vi "color_sensor.vi"() -> ()   [LabVIEW 2022 SP3]
uses:
  <vilib>/DAQmx/read.llb/DAQmx Read (Analog DBL 1Chan 1Samp).vi
  <vilib>/DAQmx/write.llb/DAQmx Write (Digital Bool 1Line 1Point).vi
  <vilib>/DAQmx/create/channels.llb/DAQmx Create Channel (DO-Digital Output).vi
  <vilib>/DAQmx/create/channels.llb/DAQmx Create Channel (AI-Voltage-Basic).vi
  <vilib>/DAQmx/miscellaneous.llb/DAQmx Fill In Error Info.vi
panel:
  out "READ VALUE":dbl
  in  "READ":tag
  in  "Blue Channel":tag
  in  "Green Channel":tag
  in  "Red Channel":tag
  in  "stop":bool
  out "green":bool
  out "blue":bool
  out "red":bool
  out "Numeric":i32
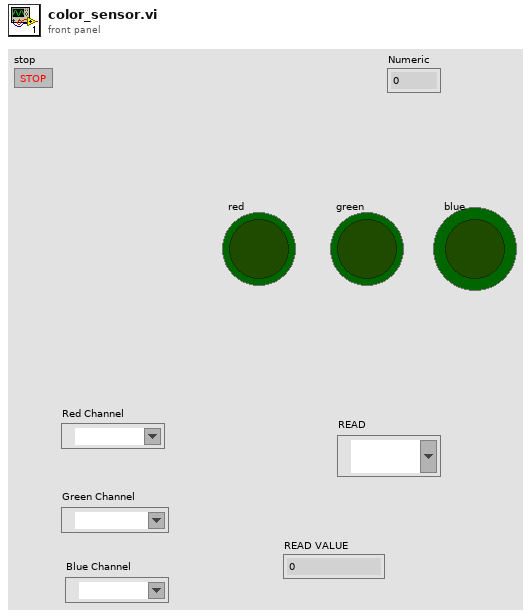
[diagram p1: front panel]
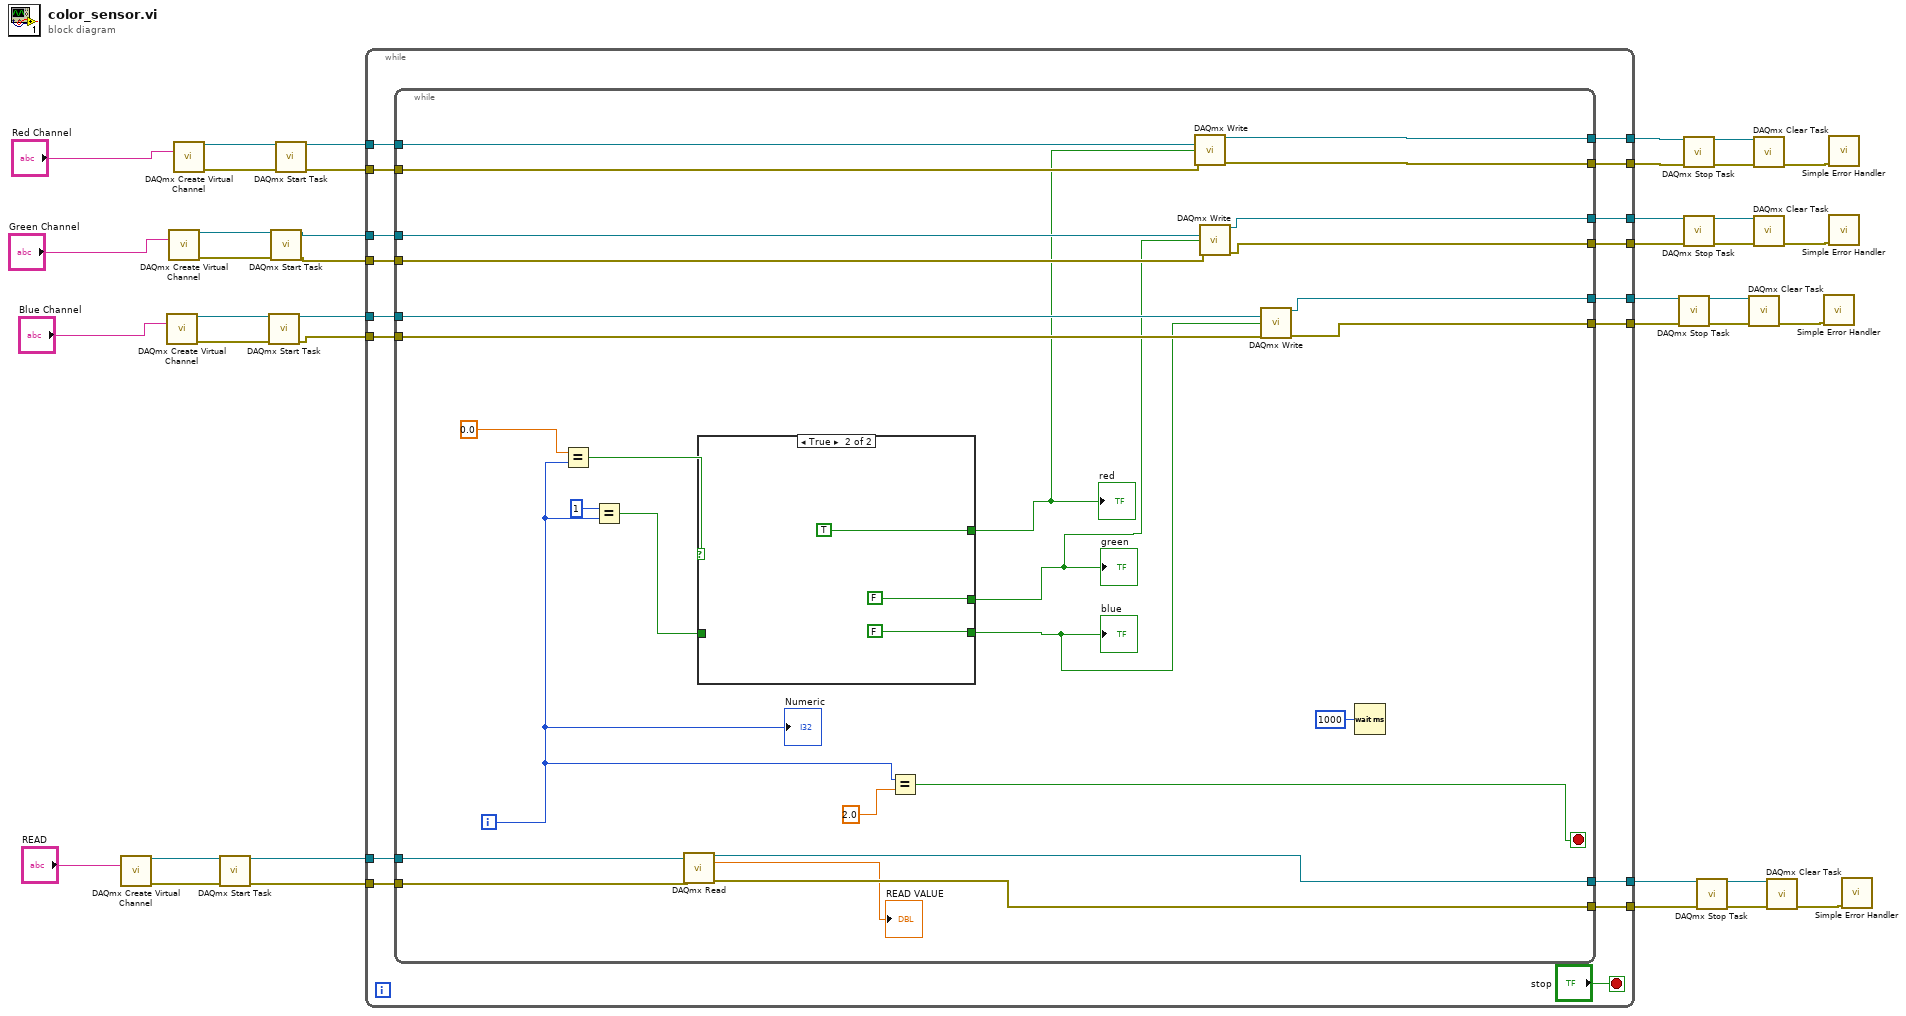
[diagram p0: block diagram]
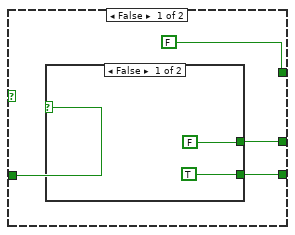
[diagram p2: hidden frame]
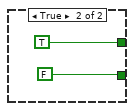
[diagram p3: hidden frame]
diagram:
  n1 = call-poly <vilib>:"DAQmx Create Virtual Channel.vi"("physical channels"="READ") -> ("task out"=w9:refnum<k21>, "error out"=w10:errorcluster)  [unwired: 13 in]
  n2 = call-poly <vilib>:"DAQmx Create Virtual Channel.vi"("lines"="Blue Channel") -> ("task out"=w21:refnum<k21>, "error out"=w22:errorcluster)  [unwired: 13 in]
  n3 = call-poly <vilib>:"DAQmx Create Virtual Channel.vi"("lines"="Green Channel") -> ("task out"=w30:refnum<k21>, "error out"=w31:errorcluster)  [unwired: 13 in]
  n4 = call-poly <vilib>:"DAQmx Create Virtual Channel.vi"("lines"="Red Channel") -> ("task out"=w39:refnum<k21>, "error out"=w40:errorcluster)  [unwired: 13 in]
  n5 = call <vilib>:"DAQmx Start Task.vi"("task/channels in"=w9, "error in"=w10) -> ("task out"=w7:refnum<k21>, "error out"=w6:errorcluster)  [unwired: 12 in]
  n6 = call <vilib>:"DAQmx Start Task.vi"("task/channels in"=w21, "error in"=w22) -> ("task out"=w20:refnum<k21>, "error out"=w19:errorcluster)  [unwired: 12 in]
  n7 = call <vilib>:"DAQmx Start Task.vi"("task/channels in"=w30, "error in"=w31) -> ("task out"=w29:refnum<k21>, "error out"=w28:errorcluster)  [unwired: 12 in]
  n8 = call <vilib>:"DAQmx Start Task.vi"("task/channels in"=w39, "error in"=w40) -> ("task out"=w38:refnum<k21>, "error out"=w37:errorcluster)  [unwired: 12 in]
  n9 = while {
    tunnel: w38 -> [w56]
    tunnel: w37 -> [w55]
    tunnel: [w54] -> w33
    tunnel: [w53] -> w32
    tunnel: w29 -> [w52]
    tunnel: w28 -> [w51]
    tunnel: [w50] -> w24
    tunnel: [w49] -> w23
    tunnel: w20 -> [w48]
    tunnel: w19 -> [w47]
    tunnel: [w46] -> w15
    tunnel: [w45] -> w14
    tunnel: w7 -> [w44]
    tunnel: w6 -> [w43]
    tunnel: [w42] -> w2
    tunnel: [w41] -> w1
    stop <- "stop" stop-if-true
    n10 = while {
      tunnel: w56 -> [w77]
      tunnel: w55 -> [w76]
      tunnel: [w75] -> w54
      tunnel: [w74] -> w53
      tunnel: w52 -> [w73]
      tunnel: w51 -> [w72]
      tunnel: [w71] -> w50
      tunnel: [w70] -> w49
      tunnel: w48 -> [w69]
      tunnel: w47 -> [w68]
      tunnel: [w67] -> w46
      tunnel: [w66] -> w45
      tunnel: w44 -> [w62]
      tunnel: w43 -> [w61]
      tunnel: [w60] -> w42
      tunnel: [w59] -> w41
      i -> [w79]
      stop <- w84 stop-if-true
      n11 = Equal?(x=0.0, y=w79) -> (x = y?=w81:bool)
      n12 = Equal?(x=1, y=w79) -> (x = y?=w80:bool)
      n13 = call-poly <vilib>:"DAQmx Read.vi"("task/channels in"=w62, "error in"=w61) -> ("task out"=w60:refnum<k21>, "data"=→"READ VALUE":dbl, "error out"=w59:errorcluster)  [unwired: 11 in]
      n14 = case shown="True" w81 {
        tunnel: [FALSE TRUE] -> w65
        tunnel: w80 -> [w89 _]
        tunnel: [w87 FALSE] -> w64
        tunnel: [w86 FALSE] -> w63
        frame False {
          n15 = case shown="False" w89 {
            tunnel: [FALSE TRUE] -> w87
            tunnel: [TRUE FALSE] -> w86
            frame False {
            }
            frame True {
            }
          }
        }
        frame True {
        }
      }
      "red" <- w65
      "blue" <- w63
      "green" <- w64
      n16 = Equal?(x=w79, y=2.0) -> (x = y?=w84:bool)
      n17 = call-poly <vilib>:"DAQmx Write.vi"("task/channels in"=w77, "data"=w65, "error in"=w76) -> ("task out"=w75:refnum<k21>, "error out"=w74:errorcluster)  [unwired: 10 in, 1 out]
      n18 = call-poly <vilib>:"DAQmx Write.vi"("task/channels in"=w73, "data"=w64, "error in"=w72) -> ("task out"=w71:refnum<k21>, "error out"=w70:errorcluster)  [unwired: 10 in, 1 out]
      n19 = call-poly <vilib>:"DAQmx Write.vi"("task/channels in"=w69, "data"=w63, "error in"=w68) -> ("task out"=w67:refnum<k21>, "error out"=w66:errorcluster)  [unwired: 10 in, 1 out]
      n20 = Wait (ms)(milliseconds to wait=u32 1000) -> ()  [unwired: 1 out]
      "Numeric" <- w79
    }
  }
  n21 = call <vilib>:"DAQmx Stop Task.vi"("task/channels in"=w15, "error in"=w14) -> ("task out"=w18:refnum<k21>, "error out"=w17:errorcluster)  [unwired: 12 in]
  n22 = call <vilib>:"DAQmx Stop Task.vi"("task/channels in"=w33, "error in"=w32) -> ("task out"=w36:refnum<k21>, "error out"=w35:errorcluster)  [unwired: 12 in]
  n23 = call <vilib>:"DAQmx Stop Task.vi"("task/channels in"=w24, "error in"=w23) -> ("task out"=w27:refnum<k21>, "error out"=w26:errorcluster)  [unwired: 12 in]
  n24 = call <vilib>:"DAQmx Stop Task.vi"("task/channels in"=w2, "error in"=w1) -> ("task out"=w5:refnum<k21>, "error out"=w4:errorcluster)  [unwired: 12 in]
  n25 = call <vilib>:"DAQmx Clear Task.vi"("task in"=w18, "error in"=w17) -> ("error out"=w16:errorcluster)  [unwired: 13 in]
  n26 = call <vilib>:"DAQmx Clear Task.vi"("task in"=w36, "error in"=w35) -> ("error out"=w34:errorcluster)  [unwired: 13 in]
  n27 = call <vilib>:"DAQmx Clear Task.vi"("task in"=w27, "error in"=w26) -> ("error out"=w25:errorcluster)  [unwired: 13 in]
  n28 = call <vilib>:"DAQmx Clear Task.vi"("task in"=w5, "error in"=w4) -> ("error out"=w3:errorcluster)  [unwired: 13 in]
  n29 = call <vilib>:"Simple Error Handler.vi"("error in (no error)"=w16) -> ()  [unwired: 4 in, 5 out]
  n30 = call <vilib>:"Simple Error Handler.vi"("error in (no error)"=w34) -> ()  [unwired: 4 in, 5 out]
  n31 = call <vilib>:"Simple Error Handler.vi"("error in (no error)"=w25) -> ()  [unwired: 4 in, 5 out]
  n32 = call <vilib>:"Simple Error Handler.vi"("error in (no error)"=w3) -> ()  [unwired: 4 in, 5 out]
